vi "Convert Array from CameraOption.vi"(1 "CAMERAOPTIONS":T1 {"VideoSystem" items=["VIDEOSYS_NTSC"=0, "VIDEOSYS_PAL"=1, "VIDEOSYS_720P60"=4, "VIDEOSYS_720P59DOT9"=12, "VIDEOSYS_720P50"=5, "VIDEOSYS_1080P30"=20, "VIDEOSYS_1080P29DOT9"=28, "VIDEOSYS_1080P25"=21, "VIDEOSYS_1080P24"=36, "VIDEOSYS_1080P23DOT9"=44, "VIDEOSYS_1080I30"=68, "VIDEOSYS_1080I29DOT9"=76, "VIDEOSYS_1080I25"=69, "VIDEOSYS_1080PSF30"=52, "VIDEOSYS_1080PSF29DOT9"=60, "VIDEOSYS_1080PSF25"=53, "VIDEOSYS_1080PSF24"=84, "VIDEOSYS_1080PSF23DOT9"=92]}) -> (0 "Array":u32[](array[numeric]))   [LabVIEW 2013, in "VRI.lvlib"]
uses:
  VRI.lvlib
  _Type Defs/PHCon CAMERAOPTIONS.ctl
  _Type Defs/PhCon VideoSystem.ctl
  _Type Defs/RGBQUAD.ctl
  _Type Defs/PHCon IMRANGE.ctl
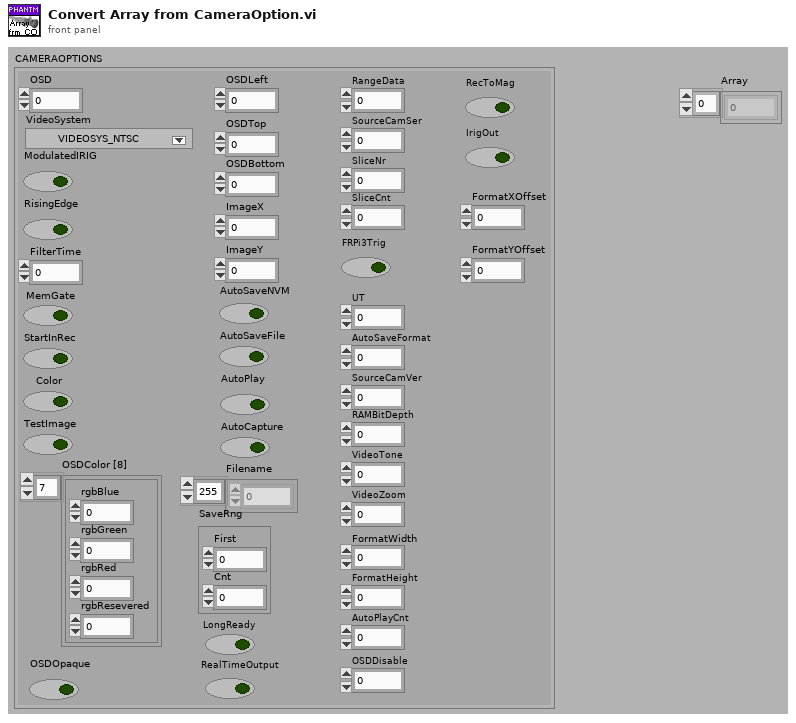
[diagram p1: front panel]
types:
  T1 = typedef "VRI.lvlib/PHCon CAMERAOPTIONS.ctl" = cluster{"OSD":u32, "VideoSystem":T2, "ModulatedIRIG":bool, "RisingEdge":bool, "FilterTime":u32, "MemGate":bool, "StartInRec":bool, "Color":bool, "TestImage":bool, "OSDColor [8]":T3[], "OSDOpaque":bool, "OSDLeft":i32, "OSDTop":i32, "OSDBottom":i32, "ImageX":i32, "ImageY":i32, "AutoSaveNVM":bool, "AutoSaveFile":bool, "AutoPlay":bool, "AutoCapture":bool, "Filename":u8[], "SaveRng":T4, "LongReady":bool, "RealTimeOutput":bool, "RangeData":u32, "SourceCamSer":u32, "SliceNr":u32, "SliceCnt":u32, "FRPi3Trig":bool, "UT":u32, "AutoSaveFormat":i8, "SourceCamVer":u32, "RAMBitDepth":u32, "VideoTone":i32, "VideoZoom":i32, "FormatWidth":i32, "FormatHeight":i32, "AutoPlayCnt":u32, "OSDDisable":u32, "RecToMag":bool, "IrigOut":bool, "FormatXOffset":i32, "FormatYOffset":i32}
  T2 = typedef "VRI.lvlib/PhCon VideoSystem.ctl" = u32
  T3 = typedef "VRI.lvlib/RGBQUAD.ctl" = cluster{"rgbBlue":u8, "rgbGreen":u8, "rgbRed":u8, "rgbResevered":u8}
  T4 = typedef "VRI.lvlib/PHCon IMRANGE.ctl" = cluster{"First":i32, "Cnt":u32}
  T5 = cluster{"OSD":u32, "VideoSystem":T2, u32, u32, "FilterTime":u32, u32, u32, u32, u32}
  T6 = cluster{u32, u32, u32, u32, u32, u32, u32, u32, u32, u32}
  T7 = cluster{u32, "RangeData":u32, "SourceCamSer":u32, "SliceNr":u32, "SliceCnt":u32, u32, "UT":u32, u32, "SourceCamVer":u32, "RAMBitDepth":u32, u32, u32, u32, u32, "AutoPlayCnt":u32, "OSDDisable":u32, u32, u32}
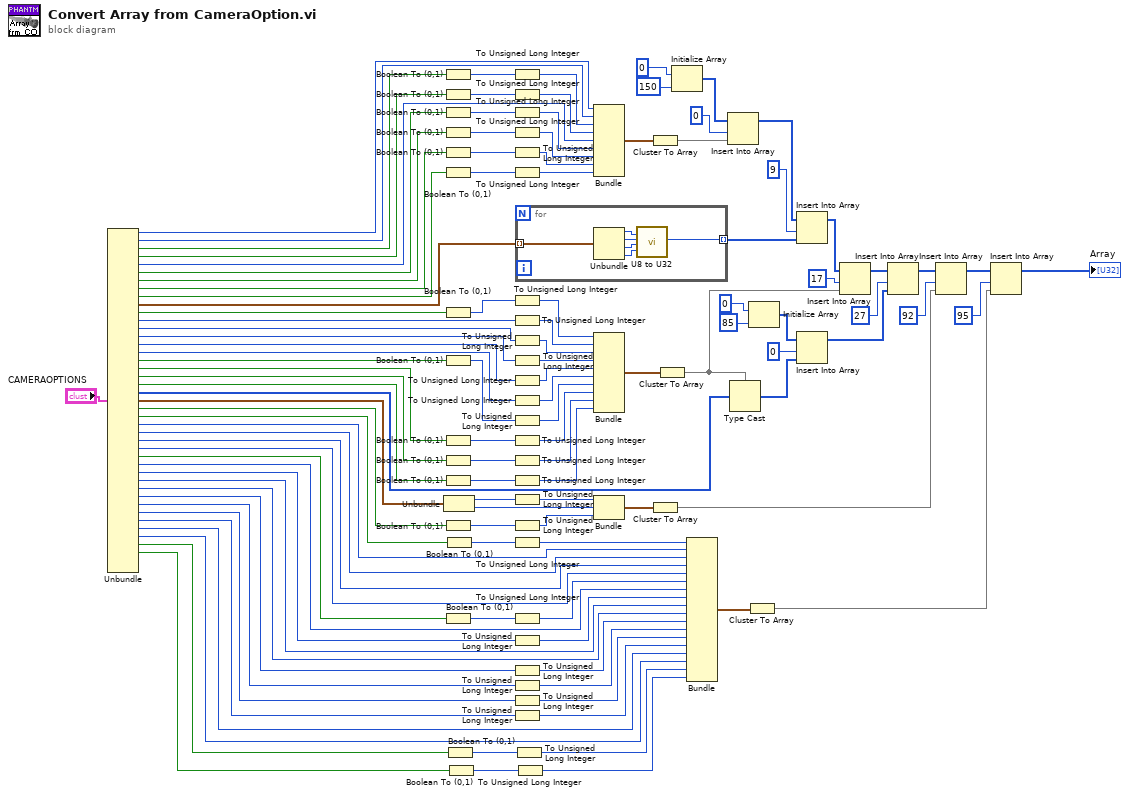
[diagram p0: block diagram]
diagram:
  n1 = Unbundle("CAMERAOPTIONS") -> ("OSD"=w94:u32, "VideoSystem"=w93:T2, "ModulatedIRIG"=w116:bool, "RisingEdge"=w115:bool, "FilterTime"=w90:u32, "MemGate"=w114:bool, "StartInRec"=w113:bool, "Color"=w112:bool, "TestImage"=w111:bool, "OSDColor [8]"=w85:T3[], "OSDOpaque"=w80:bool, "OSDLeft"=w74:i32, "OSDTop"=w72:i32, "OSDBottom"=w70:i32, "ImageX"=w68:i32, "ImageY"=w66:i32, "AutoSaveNVM"=w110:bool, "AutoSaveFile"=w109:bool, "AutoPlay"=w108:bool, "AutoCapture"=w107:bool, "Filename"=w61:u8[], "SaveRng"=w57:T4, "LongReady"=w106:bool, "RealTimeOutput"=w31:bool, "RangeData"=w28:u32, "SourceCamSer"=w27:u32, "SliceNr"=w26:u32, "SliceCnt"=w25:u32, "FRPi3Trig"=w30:bool, "UT"=w24:u32, "AutoSaveFormat"=w23:i8, "SourceCamVer"=w21:u32, "RAMBitDepth"=w20:u32, "VideoTone"=w19:i32, "VideoZoom"=w18:i32, "FormatWidth"=w17:i32, "FormatHeight"=w16:i32, "AutoPlayCnt"=w11:u32, "OSDDisable"=w10:u32, "RecToMag"=w9:bool, "IrigOut"=w8:bool)  [unwired: 2 out]
  n2 = Boolean To (0,1)(Boolean=w116) -> (0, 1=w105:i16)
  n3 = Boolean To (0,1)(Boolean=w115) -> (0, 1=w104:i16)
  n4 = Boolean To (0,1)(Boolean=w114) -> (0, 1=w103:i16)
  n5 = Boolean To (0,1)(Boolean=w113) -> (0, 1=w102:i16)
  n6 = Boolean To (0,1)(Boolean=w112) -> (0, 1=w101:i16)
  n7 = Boolean To (0,1)(Boolean=w111) -> (0, 1=w100:i16)
  n8 = Boolean To (0,1)(Boolean=w80) -> (0, 1=w81:i16)
  n9 = Boolean To (0,1)(Boolean=w110) -> (0, 1=w99:i16)
  n10 = Boolean To (0,1)(Boolean=w109) -> (0, 1=w98:i16)
  n11 = Boolean To (0,1)(Boolean=w108) -> (0, 1=w97:i16)
  n12 = Boolean To (0,1)(Boolean=w107) -> (0, 1=w96:i16)
  n13 = Boolean To (0,1)(Boolean=w106) -> (0, 1=w95:i16)
  n14 = Boolean To (0,1)(Boolean=w30) -> (0, 1=w35:i16)
  n15 = Unbundle(w57) -> ("First"=w56:i32, "Cnt"=w54:u32)
  n16 = Boolean To (0,1)(Boolean=w31) -> (0, 1=w36:i16)
  n17 = Boolean To (0,1)(Boolean=w9) -> (0, 1=w34:i16)
  n18 = Boolean To (0,1)(Boolean=w8) -> (0, 1=w33:i16)
  n19 = To Unsigned Long Integer(number=w105) -> (unsigned 32bit integer=w92:u32)
  n20 = To Unsigned Long Integer(number=w104) -> (unsigned 32bit integer=w91:u32)
  n21 = To Unsigned Long Integer(number=w103) -> (unsigned 32bit integer=w89:u32)
  n22 = To Unsigned Long Integer(number=w102) -> (unsigned 32bit integer=w88:u32)
  n23 = To Unsigned Long Integer(number=w101) -> (unsigned 32bit integer=w87:u32)
  n24 = To Unsigned Long Integer(number=w100) -> (unsigned 32bit integer=w86:u32)
  n25 = To Unsigned Long Integer(number=w81) -> (unsigned 32bit integer=w79:u32)
  n26 = To Unsigned Long Integer(number=w74) -> (unsigned 32bit integer=w73:u32)
  n27 = To Unsigned Long Integer(number=w72) -> (unsigned 32bit integer=w71:u32)
  n28 = To Unsigned Long Integer(number=w70) -> (unsigned 32bit integer=w69:u32)
  n29 = To Unsigned Long Integer(number=w68) -> (unsigned 32bit integer=w67:u32)
  n30 = To Unsigned Long Integer(number=w66) -> (unsigned 32bit integer=w65:u32)
  n31 = To Unsigned Long Integer(number=w99) -> (unsigned 32bit integer=w78:u32)
  n32 = To Unsigned Long Integer(number=w98) -> (unsigned 32bit integer=w77:u32)
  n33 = To Unsigned Long Integer(number=w97) -> (unsigned 32bit integer=w76:u32)
  n34 = To Unsigned Long Integer(number=w96) -> (unsigned 32bit integer=w75:u32)
  n35 = To Unsigned Long Integer(number=w56) -> (unsigned 32bit integer=w55:u32)
  n36 = To Unsigned Long Integer(number=w95) -> (unsigned 32bit integer=w53:u32)
  n37 = To Unsigned Long Integer(number=w36) -> (unsigned 32bit integer=w32:u32)
  n38 = To Unsigned Long Integer(number=w35) -> (unsigned 32bit integer=w29:u32)
  n39 = To Unsigned Long Integer(number=w23) -> (unsigned 32bit integer=w22:u32)
  n40 = To Unsigned Long Integer(number=w19) -> (unsigned 32bit integer=w15:u32)
  n41 = To Unsigned Long Integer(number=w18) -> (unsigned 32bit integer=w14:u32)
  n42 = To Unsigned Long Integer(number=w17) -> (unsigned 32bit integer=w13:u32)
  n43 = To Unsigned Long Integer(number=w16) -> (unsigned 32bit integer=w12:u32)
  n44 = To Unsigned Long Integer(number=w34) -> (unsigned 32bit integer=w7:u32)
  n45 = To Unsigned Long Integer(number=w33) -> (unsigned 32bit integer=w6:u32)
  n46 = for {
    tunnel: w85 -> [w123] mode=indexing
    tunnel: [w118] -> w83 mode=indexing
    n47 = Unbundle(w123) -> ("rgbBlue"=w122:u8, "rgbGreen"=w121:u8, "rgbRed"=w120:u8, "rgbResevered"=w119:u8)
    n48 = call "U8 to U32.vi"("Byte1"=w122, "Byte2"=w121, "Byte3"=w120, "Byte4"=w119) -> ("U32"=w118:u32)  [unwired: 1 in, 14 out]
  }
  n49 = Bundle("OSD"=w94, "VideoSystem"=w93, w92, w91, "FilterTime"=w90, w89, w88, w87, w86) -> (w84:T5)  [unwired: 1 out]
  n50 = Bundle(w79, w73, w71, w69, w67, w65, w78, w77, w76, w75) -> (w64:T6)  [unwired: 1 out]
  n51 = Bundle(w55, "Cnt"=w54, w53) -> (w50:cluster{u32, "Cnt":u32, u32})  [unwired: 1 out]
  n52 = Cluster To Array(cluster=w84) -> (array=w45:T2[])
  n53 = Cluster To Array(cluster=w50) -> (array=w49:u32[])
  n54 = Cluster To Array(cluster=w64) -> (array=w60:u32[])
  n55 = Initialize Array(u32 0 ("element"), 150 ("dimension size")) -> (w46:u32[])
  n56 = Bundle(w32, "RangeData"=w28, "SourceCamSer"=w27, "SliceNr"=w26, "SliceCnt"=w25, w29, "UT"=w24, w22, "SourceCamVer"=w21, "RAMBitDepth"=w20, w15, w14, w13, w12, "AutoPlayCnt"=w11, "OSDDisable"=w10, w7, w6) -> (w5:T7)  [unwired: 1 out]
  n57 = Insert Into Array(array=w46, index=0, new element=w45) -> (w44:u32[])
  n58 = Type Cast(type=w60, x=w61) -> (*(type *) &x=w38:u32[])
  n59 = Cluster To Array(cluster=w5) -> (array=w2:u32[])
  n60 = Initialize Array(u32 0 ("element"), 85 ("dimension size")) -> (w39:u32[])
  n61 = Insert Into Array(array=w44, index=9, new element=w83) -> (w63:u32[])
  n62 = Insert Into Array(array=w39, index=0, new element=w38) -> (w37:u32[])
  n63 = Insert Into Array(array=w63, index=17, new element=w60) -> (w59:u32[])
  n64 = Insert Into Array(array=w59, index=27, new element=w37) -> (w52:u32[])
  n65 = Insert Into Array(array=w52, index=92, new element=w49) -> (w3:u32[])
  n66 = Insert Into Array(array=w3, index=95, new element=w2) -> (→"Array":u32[])
